vi "climbFrontStiltLoop.vi"() -> ()   [LabVIEW 2018]
uses:
  <vilib>/Platform/TimedLoop/XDataNode/timing_clust.ctl
  <vilib>/Platform/TimedLoop/XDataNode/nitl_modes.ctl
  <vilib>/Platform/TimedLoop/XDataNode/wakeup.ctl
  <vilib>/Rock Robotics/WPI/ThirdParty/Phoenix-LabVIEW/Motor Controller/Controls/CTRE_Phoenix_MotorControl_ControlMode.ctl
  <vilib>/Rock Robotics/WPI/ThirdParty/Phoenix-LabVIEW/Motor Controller/Get/CTRE_Phoenix_MotorController_GetPulseWidthAll.vi
  <vilib>/platform/TimedLoop/XDataNode/XDataNode.xnode
  <vilib>/Platform/TimedLoop/XDataNode/XDNodeRunTimeDep.lvlib
  <vilib>/Rock Robotics/WPI/ThirdParty/Phoenix-LabVIEW/Pigeon IMU/CTRE_PigeonIMU_CalibrationMode.ctl
panel:
  in  "Power":dbl=0.2
  out "Orient Y/R/P":T1
  in  "Read Enable":T2={"Cal Status"=TRUE, "Orientation"=TRUE, "Gyro"=FALSE, "Accelerometer"=FALSE, "Quanterion"=FALSE, "Accel Mode"=enum."Linear", "Magnetometer"=FALSE, "Register Mode"=enum."Quaternion"}
  out "climbRearPosition":i32=961
  in  "New Rear Position":i32=961
  in  "New Front Position":i32
  out "Roll":dbl=0.9228515625
  out "Pitch":dbl=-11.07421875
  out "climbFrontPosition":i32=258
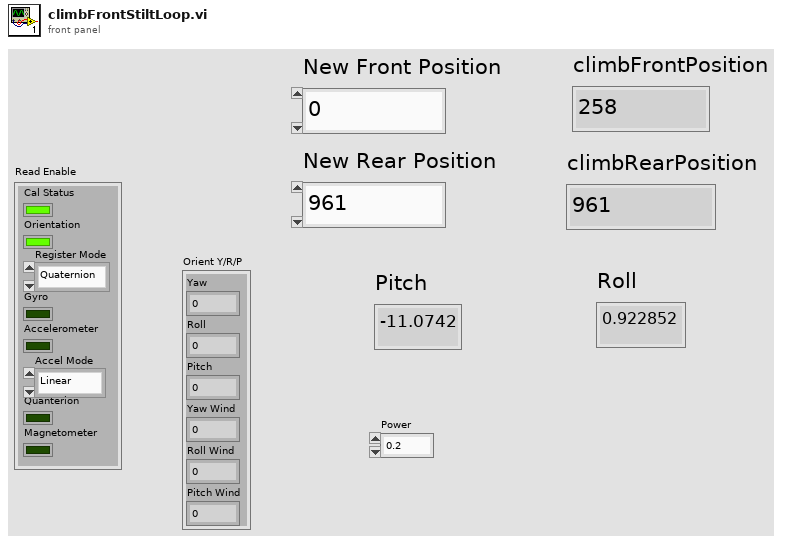
[diagram p1: front panel]
types:
  T1 = cluster{"Yaw":dbl, "Roll":dbl, "Pitch":dbl, "Yaw Wind":dbl, "Roll Wind":dbl, "Pitch Wind":dbl}
  T2 = cluster{"Cal Status":bool, "Orientation":bool, "Gyro":bool, "Accelerometer":bool, "Quanterion":bool, "Accel Mode":enum8{"Raw Data", "Linear", "Gravity"}, "Magnetometer":bool, "Register Mode":enum8{"Euler", "Quaternion"}}
  T3 = typedef "WPI_MotorControlDeviceRef.ctl" = cluster{"DeviceStatus":errorcluster, "Type":T4, "PWM":cluster{"PWM Channel":T5, "DeadBand":T6}, "CAN":cluster{"Device Number":u8, "SetOutput VI Ref":variant, "GetOutput VI Ref":variant, "Enable VI Ref":variant, "Disable VI Ref":variant, "Data":variant}, "Invert":bool, "DIO PWM":cluster{"PWM \"Enable\" Channel":T5, "DIOChannel":T7, "PWM Rate":dbl}}
  T4 = typedef "WPI_MotorControlType.ctl" = enum16{"PWM", "CAN", "DIO PWM"}
  T5 = typedef "FPGA_DIOPWMChannel.ctl" = enum8{"PWM 0", "PWM 1", "PWM 2", "PWM 3", "PWM 4", "PWM 5", "PWM 6", "PWM 7", "PWM 8", "PWM 9", "PWM MXP 0", "PWM MXP 1", "PWM MXP 2", "PWM MXP 3", "PWM MXP 4", "PWM MXP 5", "PWM MXP 6", "PWM MXP 7", "PWM MXP 8", "PWM MXP 9", "Invalid"}
  T6 = typedef "WPI_PWMDeadband.ctl" = cluster{"Name":string, "maxPositivePwm":i32, "minPositivePwm":i32, "centerPwm":i32, "maxNegativePwm":i32, "minNegativePwm":i32, "angularRange":u16}
  T7 = typedef "FPGA_DIOChannel.ctl" = enum8{"DIO 0", "DIO 1", "DIO 2", "DIO 3", "DIO 4", "DIO 5", "DIO 6", "DIO 7", "DIO 8", "DIO 9", "DIO MXP 0", "DIO MXP 1", "DIO MXP 2", "DIO MXP 3", "DIO MXP 4", "DIO MXP 5", "DIO MXP 6", "DIO MXP 7", "DIO MXP 8", "DIO MXP 9", "DIO MXP 10", "DIO MXP 11", "DIO MXP 12", "DIO MXP 13", "DIO MXP 14", "DIO MXP 15", "SPI Port CS1", "SPI Port CS2", "SPI Port CS3", "SPI Port MISO", "SPI Port MOSI", "Invalid"}
  T8 = typedef "CTRE_PigeonIMU_DeviceRef.ctl" = cluster{"DeviceStatus":errorcluster, "Device Number":u8, "Type":T9, "Device ID":u32, "Handle":u64, "UsageFrame":u32, "Library Path":path}
  T9 = typedef "CTRE_PigeonIMU_ConnectionType.ctl" = u32
  T10 = typedef "ImuDevRef.ctl" = cluster{"I2CDevRef":T11, "Valid Cal File?":bool}
  T11 = typedef "WPI_I2CDevRef.ctl" = cluster{"DevStatus":errorcluster, "Device Address":u8, "Handle":i32, "I2C Bus":T12}
  T12 = typedef "i2c_bus.ctl" = enum16{"I2C On-Board", "I2C MXP", "Invalid"}
  T13 = typedef "XDNodeRunTimeDep.lvlib/timing_clust.ctl" = cluster{"Expected End [f-1]":u64, "Actual End [f-1]":u64, "Finished Late? [f-1]":bool, "Expected End [i-1]":u64, "Actual End [i-1]":u64, "Finished Late? [i-1]":bool, "Expected Start [i]":u64, "Actual Start [i]":u64, "Expected Start [f]":u64, "Actual Start [f]":u64, "Source Name":string, "Structure Name":string, "Period":i64, "Deadline":i64, "Offset":i64, "Start":i64, "Priority":i32, "Timeout":i32, "Mode":T14, "Wakeup Reason":T15, "Error":errorcluster, "Source Type":string, "Secondary Source Type":string, "Global End Time":u64, "Global Start Time":u64, "Frame Duration":u64, "Iteration Duration":u64, "Assigned CPU":i32, "I/O Scan Engine Mode":u32}
  T14 = typedef "XDNodeRunTimeDep.lvlib/nitl_modes.ctl" = enum32{"No Change", "Process missed periods, maintain original phase", "Discard missed periods, maintain original phase", "Process missed periods, ignore original phase", "Discard missed periods, ignore original phase"}
  T15 = typedef "XDNodeRunTimeDep.lvlib/wakeup.ctl" = enum32{"Normal", "Aborted", "Asynchronous wakeup", "Timing source error", "Timed loop error", "Timeout"}
  T16 = typedef "CTRE_Phoenix_MotorControl_ControlMode.ctl" = u16
  T17 = typedef "CTRE_PigeonIMU_CalibrationMode.ctl" = u16
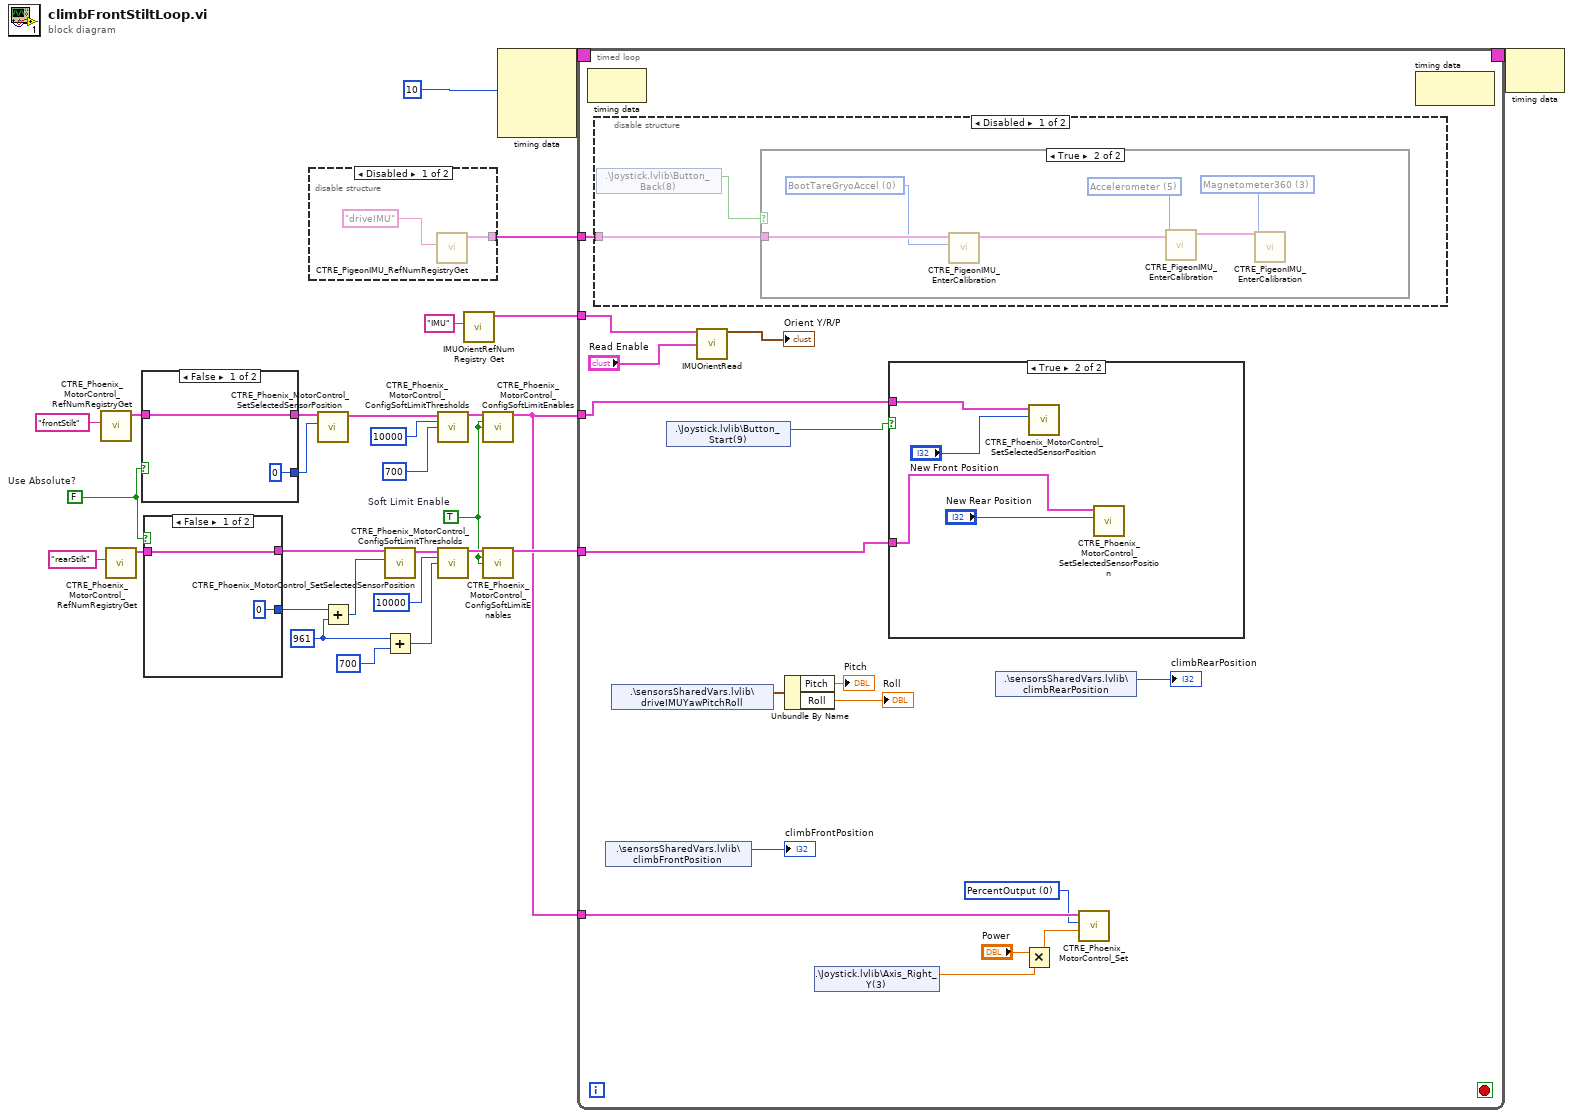
[diagram p0: block diagram]
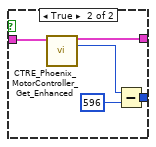
[diagram p3: hidden frame]
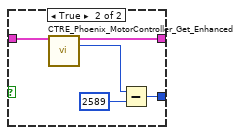
[diagram p4: hidden frame]
diagram:
  w1 = TRUE  # Soft Limit Enable
  w14 = FALSE  # Use Absolute?
  w11 = 961 ("y")
  n1 = call <vilib>:"CTRE_Phoenix_MotorControl_RefNumRegistryGet.vi"("refnum name"="frontStilt") -> ("PhoenixMotorControlDevRef"=w21:T3)  [unwired: 9 in, 1 out]
  n2 = call <vilib>:"CTRE_Phoenix_MotorControl_RefNumRegistryGet.vi"("refnum name"="rearStilt") -> ("PhoenixMotorControlDevRef"=w17:T3)  [unwired: 9 in, 1 out]
  n3 = case shown="False" w14 {
    tunnel: w21 -> [w30 w36]
    tunnel: [w30 w33] -> w20
    tunnel: [0 w32] -> w19
    frame False {
    }
    frame True {
      n4 = call-poly <vilib>:"CTRE_Phoenix_MotorController_Get_Enhanced.vi"("PhoenixMotorControlDevRef"=w36) -> ("PhoenixMotorControlDevRef"=w33:T3, "Pulse Width Position"=w35:i32)  [unwired: 9 in, 4 out]
      n5 = Subtract(x=w35, y=2589) -> (x-y=w32:i32)
    }
  }
  n6 = case shown="False" w14 {
    tunnel: [0 w41] -> w18
    tunnel: w17 -> [w37 w40]
    tunnel: [w37 w39] -> w16
    frame False {
    }
    frame True {
      n7 = call-poly <vilib>:"CTRE_Phoenix_MotorController_Get_Enhanced.vi"("PhoenixMotorControlDevRef"=w40) -> ("PhoenixMotorControlDevRef"=w39:T3, "Pulse Width Position"=w42:i32)  [unwired: 9 in, 4 out]
      n8 = Subtract(x=w42, y=596) -> (x-y=w41:i32)
    }
  }
  n9 = disable-structure shown="Disabled" {
    disable-tunnel: [w44 _] -> w24
    frame Disabled {
      n10 = call <vilib>:"CTRE_PigeonIMU_RefNumRegistryGet.vi"("refnum name"="driveIMU") -> ("PigeonIMUDevRef"=w44:T8)  [unwired: 9 in, 1 out]
    }
    frame Enabled {
    }
  }
  n11 = call <vilib>:"CTRE_Phoenix_MotorControl_SetSelectedSensorPosition.vi"("New Sensor Position"=w19, "PhoenixMotorControlDevRef"=w20) -> ("PhoenixMotorControlDevRef"=w13:T3)  [unwired: 8 in, 1 out]
  n12 = Add(x=w18, y=w11) -> (x+y=w15:i32)
  n13 = call <vilib>:"CTRE_Phoenix_MotorControl_SetSelectedSensorPosition.vi"("New Sensor Position"=w15, "PhoenixMotorControlDevRef"=w16) -> ("PhoenixMotorControlDevRef"=w6:T3)  [unwired: 8 in, 1 out]
  n14 = Add(x=w11, y=700) -> (x+y=w10:i32)
  n15 = call <vilib>:"CTRE_Phoenix_MotorControl_ConfigSoftLimitThresholds.vi"("PhoenixMotorControlDevRef"=w13, "Forward Soft Limit"=10000, "Reverse Soft Limit"=700) -> ("PhoenixMotorControlDevRef"=w3:T3)  [unwired: 11 in, 1 out]
  n16 = call <vilib>:"CTRE_Phoenix_MotorControl_ConfigSoftLimitThresholds.vi"("PhoenixMotorControlDevRef"=w6, "Forward Soft Limit"=10000, "Reverse Soft Limit"=w10) -> ("PhoenixMotorControlDevRef"=w5:T3)  [unwired: 11 in, 1 out]
  n17 = call <userlib>:"IMUOrientRefNum Registry Get.vi"("refnum name"="IMU") -> ("IMUDevRef out"=w22:T10)  [unwired: 9 in, 1 out]
  n18 = call <vilib>:"CTRE_Phoenix_MotorControl_ConfigSoftLimitEnables.vi"("PhoenixMotorControlDevRef"=w3, "Forward Soft Limit Enable"=w1, "Reverse Soft Limit Enable"=w1) -> ("PhoenixMotorControlDevRef"=w2:T3)  [unwired: 11 in, 1 out]
  n19 = call <vilib>:"CTRE_Phoenix_MotorControl_ConfigSoftLimitEnables.vi"("PhoenixMotorControlDevRef"=w5, "Forward Soft Limit Enable"=w1, "Reverse Soft Limit Enable"=w1) -> ("PhoenixMotorControlDevRef"=w4:T3)  [unwired: 11 in, 1 out]
  n20 = node-c288(i64 10 ("Period")) -> (w28:T13)  [unwired: 3 in]
  n21 = timed-loop {
    timing: w28 -> [_]
    timing-out: [_] -> w27
    tunnel: w2 -> [w52]
    tunnel: w4 -> [w51]
    tunnel: w24 -> [w56]
    tunnel: w22 -> [w55]
    tunnel: w2 -> [w50]
    stop <- _ stop-if-true
    w49 = T16 0 items=["PercentOutput"=0, "Position"=1, "Velocity"=2, "Current"=3, "Follower"=5, "MotionProfile"=6, "MotionMagic"=7, "MotionProfileArc"=10, "Disabled"=15] ("Control Mode")
    n22 = node-c288() -> ()  [unwired: 1 in, 1 out]
    n23 = disable-structure shown="Disabled" {
      disable-tunnel: w56 -> [w63 _]
      frame Disabled {
        n24 = shared-variable ".\\Joystick.lvlib\\Button_Back(8)"() -> (w64:bool)  [unwired: 1 in, 1 out]
        n25 = case shown="True" w64 {
          tunnel: w63 -> [_ w70]
          frame False {
          }
          frame True {
            w66 = T17 3 items=["BootTareGryoAccel"=0, "Temperature"=1, "Magnetometer12Pt"=2, "Magnetometer360"=3, "Accelerometer"=5] ("CalibrationMode")
            w67 = T17 5 items=["BootTareGryoAccel"=0, "Temperature"=1, "Magnetometer12Pt"=2, "Magnetometer360"=3, "Accelerometer"=5] ("CalibrationMode")
            w69 = T17 0 items=["BootTareGryoAccel"=0, "Temperature"=1, "Magnetometer12Pt"=2, "Magnetometer360"=3, "Accelerometer"=5] ("CalibrationMode")
            n26 = call <vilib>:"CTRE_PigeonIMU_EnterCalibration.vi"("CalibrationMode"=w69, "PigeonIMUDevRef"=w70) -> ("PigeonIMUDevRef"=w65:T8)  [unwired: 8 in, 1 out]
            n27 = call <vilib>:"CTRE_PigeonIMU_EnterCalibration.vi"("CalibrationMode"=w67, "PigeonIMUDevRef"=w65) -> ("PigeonIMUDevRef"=w68:T8)  [unwired: 8 in, 1 out]
            n28 = call <vilib>:"CTRE_PigeonIMU_EnterCalibration.vi"("CalibrationMode"=w66, "PigeonIMUDevRef"=w68) -> ()  [unwired: 8 in, 2 out]
          }
        }
      }
      frame Enabled {
      }
    }
    n29 = shared-variable ".\\sensorsSharedVars.lvlib\\climbFrontPosition"() -> (→"climbFrontPosition":i32)  [unwired: 1 in, 1 out]
    n30 = shared-variable ".\\sensorsSharedVars.lvlib\\driveIMUYawPitchRoll"() -> (w61:cluster{"Yaw":dbl, "Pitch":dbl, "Roll":dbl})  [unwired: 1 in, 1 out]
    n31 = shared-variable ".\\Joystick.lvlib\\Button_Start(9)"() -> (w58:bool)  [unwired: 1 in, 1 out]
    n32 = call <userlib>:"IMUOrientRead.vi"("IMU Dev Ref"=w55, "Read Enable"="Read Enable") -> ("Orient Y/R/P"=→"Orient Y/R/P":T1)  [unwired: 6 in, 7 out]
    n33 = Unbundle By Name(w61) -> ("Pitch"=→"Pitch":dbl, "Roll"=→"Roll":dbl)
    n34 = shared-variable ".\\Joystick.lvlib\\Axis_Right_Y(3)"() -> (w48:dbl)  [unwired: 1 in, 1 out]
    n35 = case shown="True" w58 {
      tunnel: w52 -> [_ w74]
      tunnel: w51 -> [_ w71]
      frame False {
      }
      frame True {
        n36 = call <vilib>:"CTRE_Phoenix_MotorControl_SetSelectedSensorPosition.vi"("New Sensor Position"="New Front Position", "PhoenixMotorControlDevRef"=w74) -> ()  [unwired: 8 in, 2 out]
        n37 = call <vilib>:"CTRE_Phoenix_MotorControl_SetSelectedSensorPosition.vi"("New Sensor Position"="New Rear Position", "PhoenixMotorControlDevRef"=w71) -> ()  [unwired: 8 in, 2 out]
      }
    }
    n38 = shared-variable ".\\sensorsSharedVars.lvlib\\climbRearPosition"() -> (→"climbRearPosition":i32)  [unwired: 1 in, 1 out]
    n39 = Multiply(x="Power", y=w48) -> (x*y=w47:dbl)
    n40 = call <vilib>:"CTRE_Phoenix_MotorControl_Set.vi"("Output"=w47, "Control Mode"=w49, "PhoenixMotorControlDevRef"=w50) -> ()  [unwired: 7 in, 2 out]
    n41 = node-c288() -> ()  [unwired: 1 in, 1 out]
  }
  n42 = node-c288(w27) -> ()  [unwired: 1 out]
